vi "dashboard_logger.vi"(11 "data occurrence":refnum<k4>) -> ()   [LabVIEW 2011]
uses:
  drivetrain/gear_shift_state.ctl
  gun/gun_motor_state.ctl
  dashboard_globals.vi
panel:
  in  "quit logger":bool
  in  "Logger Enable":bool
  in  "Subsystems To Log":cluster{"Log Points":bool, "Name":string}[](array[cluster])=[{"Log Points"=FALSE, "Name"="drivetrain"}, {"Log Points"=FALSE, "Name"="gun_rt_fast"}, {"Log Points"=FALSE, "Name"="gun_rt_slow"}, {"Log Points"=FALSE, "Name"="joe_johnson"}, {"Log Points"=FALSE, "Name"="roller"}, {"Log Points"=TRUE, "Name"="system"}]
  # "off"
  # "on"
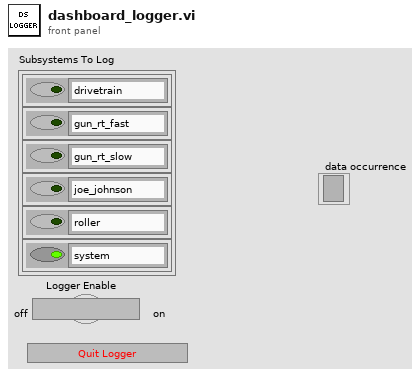
[diagram p1: front panel]
types:
  T1 = typedef "gun_motor_state.ctl" = enum16{"Hold Power", "Hold Speed", "Hold Distance", "Stop"}
  T2 = typedef "gear_shift_state.ctl" = enum16{"low", "high"}
  T3 = enum16{"open", "replace", "create", "open or create", "replace or create", "replace or create with confirmation"}
  T4 = cluster{"Subsystems To Log[0]":cluster{"Log Points":bool, "Name":string}, "Subsystems To Log[1]":cluster{"Log Points":bool, "Name":string}, "Subsystems To Log[2]":cluster{"Log Points":bool, "Name":string}, "Subsystems To Log[3]":cluster{"Log Points":bool, "Name":string}, "Subsystems To Log[4]":cluster{"Log Points":bool, "Name":string}, "Subsystems To Log[5]":cluster{"Log Points":bool, "Name":string}}
  T5 = typedef "dashboard_data_gun_fast.ctl" = cluster{"speed_setpoint":dbl, "speed_sensor":dbl, "gun_power":dbl, "gun_control_mode":T1, "gun_tracking_mode":T6}
  T6 = typedef "gun_tracking_mode.ctl" = enum16{"manual_aim", "auto_aim_camera", "preset_center_field", "preset_right_pocket", "preset_left_pocket", "align_center", "align_center_backwards", "auto_aim_key", "align_fold", "auton_custom", "preset_pass", "auto_aim_auton"}
  T7 = typedef "gun_rt_slow_upstream_data.ctl" = cluster{"turret":cluster{"turret_analog":dbl, "turret_angle":dbl, "turret_motor":dbl, "turret_idg_state":T8}, "hood":cluster{"hood_analog":dbl, "hood_angle":dbl, "hood_motor":dbl, "hood_idg_state":T8}}
  T8 = typedef "idg_trust_t.ctl" = enum16{"fault_move", "fault_high", "fault_low", "out_high", "out_low", "trust"}
  T9 = typedef "dashboard_data_drivetrain.ctl" = cluster{"left":cluster{"request":dbl, "enc_speed":dbl}, "right":cluster{"request":dbl, "enc_speed":dbl}, "gear shift state":T2, "gear shift internal state":T10}
  T10 = typedef "gear_internal_shift_state.ctl" = enum16{"low", "high", "low_peak", "high_peak"}
  T11 = typedef "roller_internal_state.ctl" = enum16{"idle", "bump", "full", "fire_intermediate", "fire_finish", "fire_entry", "fire_end", "fire_recover"}
  T12 = typedef "roller_user_state.ctl" = enum16{"off", "collect", "blow", "force suck"}
  T13 = typedef "joe_johnson_state.ctl" = enum16{"fold", "down", "up", "ramp", "bridge_lift", "manual", "ramp_stay"}
  T14 = cluster{"gun_fast":T5, "gun_slow":T7, "drivetrain_data":T9, "roller data":cluster{"roller internal state":T11, "roller user state":T12, "sws":cluster{"r_sw_b1":bool, "r_sw_b2":bool, "r_sw_b3":bool, "r_sw_gun":bool, "r_sw_low":bool}}, "joe_johnson_data":cluster{"analog":dbl, "input":dbl, "joe_johnson_state":T13, "idg_state":T8}}
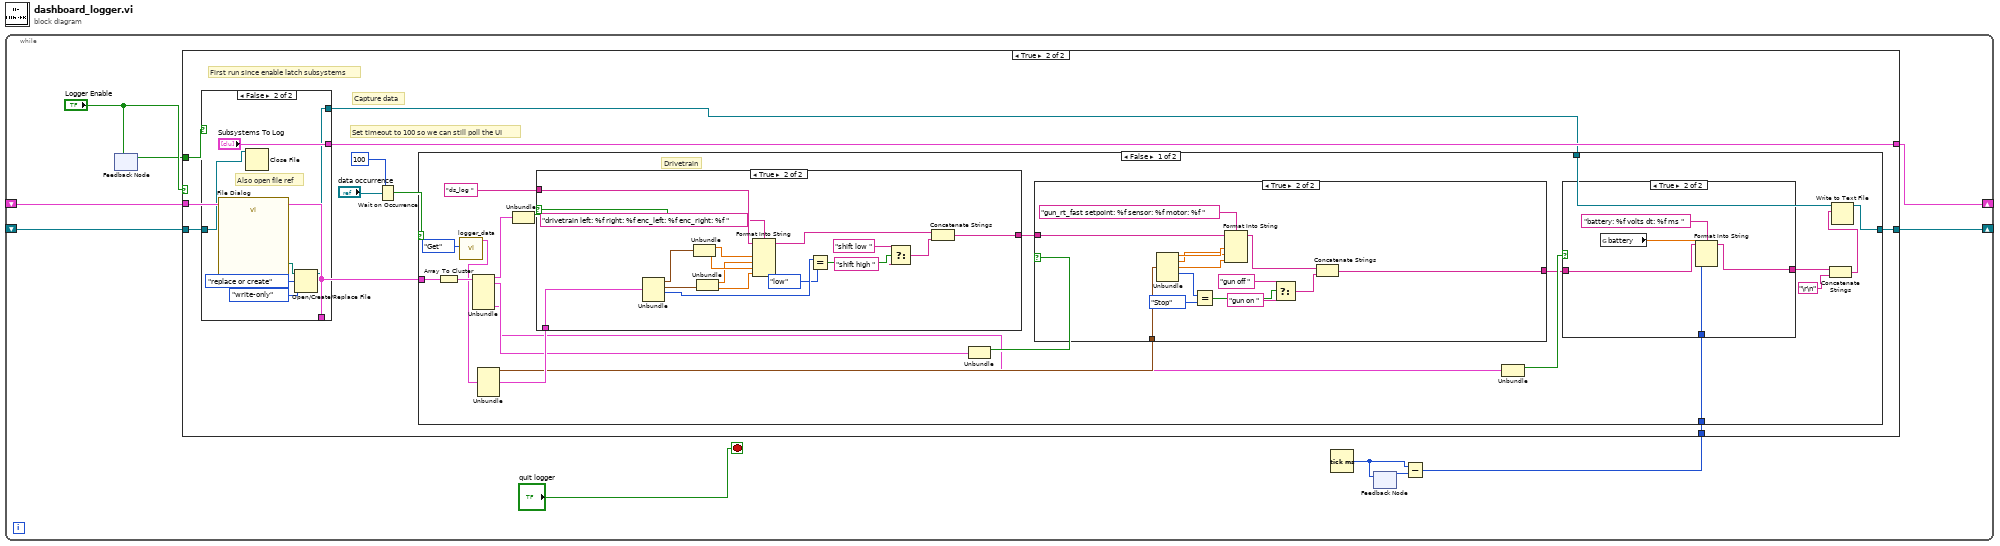
[diagram p0: block diagram]
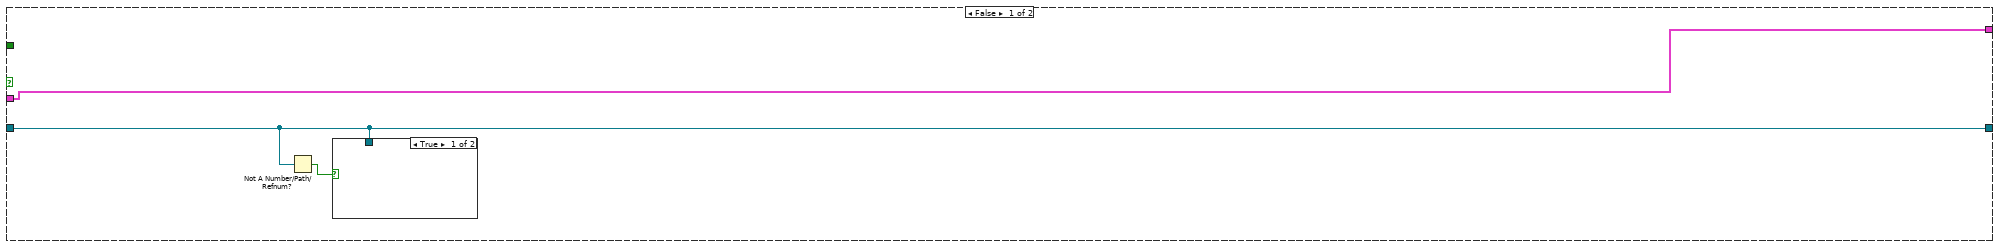
[diagram p2: hidden frame]
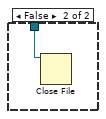
[diagram p3: hidden frame]
diagram:
  n1 = while {
    shift-right: [w9] -> _
    shift-left: _ -> [w7]
    shift-right: [w4] -> _
    shift-left: _ -> [w5]
    stop <- "quit logger" stop-if-true
    n2 = feedback-in #1("Logger Enable") -> ()
    n3 = feedback #1() -> (w8:bool)  [unwired: 1 in]
    n4 = Tick Count (ms)() -> (millisecond timer value=w3:u32)
    n5 = feedback-in #2(w3) -> ()
    n6 = feedback #2() -> (w2:u32)  [unwired: 1 in]
    n7 = Subtract(x=w3, y=w2) -> (x-y=w1:u32)
    n8 = case shown="True" "Logger Enable" {
      tunnel: [w13 w22] -> w9
      tunnel: w8 -> [_ w21]
      tunnel: w7 -> [w13 w19]
      tunnel: w5 -> [w12 w18]
      tunnel: [w12 w16] -> w4
      tunnel: w1 -> [_ w15]
      frame False {
        n9 = Not A Number/Path/Refnum?(number/path/refnum=w12) -> (NaN/Path/Refnum?=w11:bool)
        n10 = case shown="True" w11 {
          tunnel: w12 -> [_ w14]
          frame True {
          }
          frame False {
            n11 = Close File(refnum=w14) -> ()  [unwired: 1 in, 2 out]
          }
        }
      }
      frame True {
        # "First run since enable latch subsystems"
        # "Set timeout to 100 so we can still poll the UI"
        # "Capture data"
        n12 = case shown="False" w21 {
          tunnel: [w87 "Subsystems To Log"] -> w22
          tunnel: w19 -> [w87 _]
          tunnel: w18 -> [w86 w88]
          tunnel: [w86 w91] -> w17
          frame True {
          }
          frame False {
            # "Also open file ref"
            n13 = call "File Dialog"() -> ("selected path"=w92:path)  [unwired: 12 in, 3 out]
            n14 = Close File(refnum=w88) -> ()  [unwired: 1 in, 2 out]
            n15 = Open/Create/Replace File(file path (use dialog)=w92, operation (0:open)=T3."replace or create", access (0:read/write)=enum16{"read/write", "read-only", "write-only"}."write-only") -> (refnum out=w91:refnum<file>)  [unwired: 3 in, 2 out]
          }
        }
        n16 = Wait on Occurrence(2:"data occurrence", 3:100 ("ms timeout (-1)")) -> (0:w20:bool)  [unwired: 1 in]
        n17 = case shown="False" w20 {
          tunnel: w19 -> [w45 _]
          tunnel: w17 -> [w33 w85]
          tunnel: [w32 w85] -> w16
          tunnel: w15 -> [w25 _]
          frame False {
            # "Drivetrain"
            n18 = Array To Cluster(array=w45) -> (cluster=w44:T4)
            n19 = call "logger_data.vi"("data_store_mode"=enum16{"Set", "Get"}."Get") -> ("dashboard_data_out"=w40:T14)  [unwired: 10 in]
            n20 = Unbundle(w44) -> ("Subsystems To Log[0]"=w43:cluster{"Log Points":bool, "Name":string}, "Subsystems To Log[1]"=w37:cluster{"Log Points":bool, "Name":string}, "Subsystems To Log[5]"=w29:cluster{"Log Points":bool, "Name":string})  [unwired: 3 out]
            n21 = Unbundle(w40) -> ("gun_fast"=w35:T5, "drivetrain_data"=w38:T9)  [unwired: 3 out]
            n22 = Unbundle(w43) -> ("Log Points"=w42:bool)  [unwired: 1 out]
            n23 = case shown="True" w42 {
              tunnel: "ds_log " -> [w67 w84]
              tunnel: w38 -> [_ w82]
              tunnel: [w67 w68] -> w34
              frame False {
              }
              frame True {
                n24 = Unbundle(w82) -> ("left"=w81:cluster{"request":dbl, "enc_speed":dbl}, "right"=w78:cluster{"request":dbl, "enc_speed":dbl}, "gear shift state"=w75:T2)  [unwired: 1 out]
                n25 = Unbundle(w81) -> ("request"=w80:dbl, "enc_speed"=w79:dbl)
                n26 = Unbundle(w78) -> ("request"=w77:dbl, "enc_speed"=w76:dbl)
                n27 = Format Into String(format string="drivetrain left: %f right: %f enc_left: %f enc_right: %f ", initial string=w84, w80, w77, w79, w76) -> (resulting string=w70:string)  [unwired: 1 in, 1 out]
                n28 = Equal?(x=w75, y=gear_shift_state."low") -> (x = y?=w73:bool)
                n29 = Select(t="shift low ", s=w73, f="shift high ") -> (s? t:f=w69:string)
                n30 = Concatenate Strings(w70, w69) -> (w68:string)
              }
            }
            n31 = Unbundle(w37) -> ("Log Points"=w36:bool)  [unwired: 1 out]
            n32 = case shown="True" w36 {
              tunnel: w35 -> [_ w66]
              tunnel: w34 -> [w52 w64]
              tunnel: [w52 w53] -> w27
              frame False {
              }
              frame True {
                n33 = Unbundle(w66) -> ("speed_setpoint"=w63:dbl, "speed_sensor"=w62:dbl, "gun_power"=w61:dbl, "gun_control_mode"=w55:T1)  [unwired: 1 out]
                n34 = Equal?(x=w55, y=gun_motor_state."Stop") -> (x = y?=w60:bool)
                n35 = Format Into String(format string="gun_rt_fast setpoint: %f sensor: %f motor: %f ", initial string=w64, w63, w62, w61) -> (resulting string=w56:string)  [unwired: 1 in, 1 out]
                n36 = Select(t="gun off ", s=w60, f="gun on ") -> (s? t:f=w57:string)
                n37 = Concatenate Strings(w56, w57) -> (w53:string)
              }
            }
            n38 = Unbundle(w29) -> ("Log Points"=w28:bool)  [unwired: 1 out]
            n39 = case shown="True" w28 {
              tunnel: w27 -> [w46 w51]
              tunnel: [w46 w50] -> w26
              tunnel: w25 -> [_ w47]
              frame False {
              }
              frame True {
                n40 = global read "dashboard_globals.vi" "battery"() -> (w48:dbl)
                n41 = Format Into String(format string="battery: %f volts dt: %f ms ", initial string=w51, w48, w47) -> (resulting string=w50:string)  [unwired: 1 in, 1 out]
              }
            }
            n42 = Concatenate Strings(w26, "\r\n") -> (w31:string)
            n43 = Write to Text File(file (use dialog)=w33, text=w31) -> (refnum out=w32:refnum<file>)  [unwired: 2 in, 2 out]
          }
          frame True {
            # "Timed out - Wait till the next loop"
          }
        }
      }
    }
  }
